vi "fastseq_set_orders.vi"(0 "FPGA VI Reference In":T2, 1 "pulse length":u16, 2 "divider":u32, 3 "sample count":u16, 4 "Enum":T1(ring)) -> (5 "FPGA VI Reference Out":T2)   [LabVIEW 2013]
uses:
  fpga-bitfile-ref.ctl
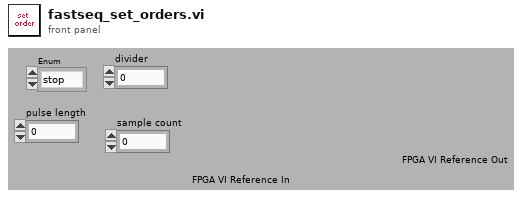
[diagram p1: front panel]
types:
  T1 = enum16{"stop", "set divider", "unset ramp mode", "unset stop count", "set pulse lenght", "set ramp", "start"}
  T2 = typedef "fpga-bitfile-ref.ctl" = refnum<k20>
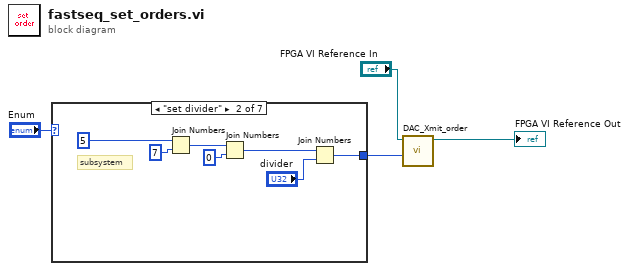
[diagram p0: block diagram]
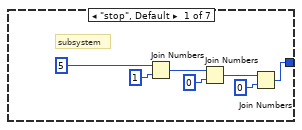
[diagram p2: hidden frame]
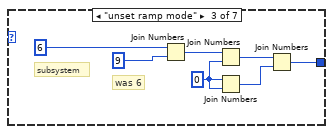
[diagram p3: hidden frame]
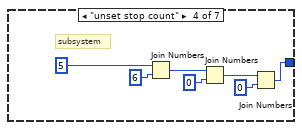
[diagram p4: hidden frame]
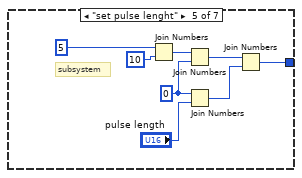
[diagram p5: hidden frame]
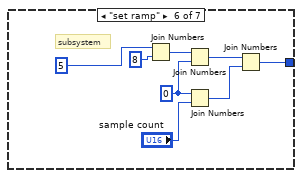
[diagram p6: hidden frame]
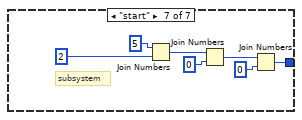
[diagram p7: hidden frame]
diagram:
  n1 = case shown="\"set divider\"" "Enum" {
    tunnel: [w5 w12 w19 w26 w33 w41 w49] -> w4
    frame "stop", Default {
      # "subsystem"
      n2 = Join Numbers(hi=u8 5, lo=u8 1) -> ((hi.lo)=w11:u16)
      n3 = Join Numbers(hi=w11, lo=u16 0) -> ((hi.lo)=w9:u32)
      n4 = Join Numbers(hi=w9, lo=u32 0) -> ((hi.lo)=w5:u64)
    }
    frame "set divider" {
      # "subsystem"
      n5 = Join Numbers(hi=u8 5, lo=u8 7) -> ((hi.lo)=w18:u16)
      n6 = Join Numbers(hi=w18, lo=u16 0) -> ((hi.lo)=w16:u32)
      n7 = Join Numbers(hi=w16, lo="divider") -> ((hi.lo)=w12:u64)
    }
    frame "unset ramp mode" {
      w20 = u16 0 ("lo")
      # "was 6"
      # "subsystem"
      n8 = Join Numbers(hi=u8 6, lo=u8 9) -> ((hi.lo)=w25:u16)
      n9 = Join Numbers(hi=w25, lo=w20) -> ((hi.lo)=w23:u32)
      n10 = Join Numbers(hi=w20, lo=w20) -> ((hi.lo)=w21:u32)
      n11 = Join Numbers(hi=w23, lo=w21) -> ((hi.lo)=w19:u64)
    }
    frame "unset stop count" {
      # "subsystem"
      n12 = Join Numbers(hi=u8 5, lo=u8 6) -> ((hi.lo)=w32:u16)
      n13 = Join Numbers(hi=w32, lo=u16 0) -> ((hi.lo)=w30:u32)
      n14 = Join Numbers(hi=w30, lo=u32 0) -> ((hi.lo)=w26:u64)
    }
    frame "set pulse lenght" {
      w34 = u16 0 ("lo")
      # "subsystem"
      n15 = Join Numbers(hi=u8 5, lo=u8 10) -> ((hi.lo)=w40:u16)
      n16 = Join Numbers(hi=w40, lo=w34) -> ((hi.lo)=w38:u32)
      n17 = Join Numbers(hi=w34, lo="pulse length") -> ((hi.lo)=w36:u32)
      n18 = Join Numbers(hi=w38, lo=w36) -> ((hi.lo)=w33:u64)
    }
    frame "set ramp" {
      w42 = u16 0 ("lo")
      # "subsystem"
      n19 = Join Numbers(hi=u8 5, lo=u8 8) -> ((hi.lo)=w48:u16)
      n20 = Join Numbers(hi=w48, lo=w42) -> ((hi.lo)=w46:u32)
      n21 = Join Numbers(hi=w42, lo="sample count") -> ((hi.lo)=w44:u32)
      n22 = Join Numbers(hi=w46, lo=w44) -> ((hi.lo)=w41:u64)
    }
    frame "start" {
      # "subsystem"
      n23 = Join Numbers(hi=u8 5, lo=u8 2) -> ((hi.lo)=w55:u16)
      n24 = Join Numbers(hi=w55, lo=u16 0) -> ((hi.lo)=w53:u32)
      n25 = Join Numbers(hi=w53, lo=u32 0) -> ((hi.lo)=w49:u64)
    }
  }
  n26 = call "DAC_Xmit_order.vi"("Order in"=w4, "FPGA VI Reference In"="FPGA VI Reference In") -> ("FPGA VI Reference Out"=→"FPGA VI Reference Out":T2)  [unwired: 9 out]
